vi "Time Countdown BAP4B.vi"(0 "Before Loop":i64, 1 "system state in":T1={"last light state"=enum."init", "light state"=enum."init", "state time (ms)"=0, "current time (ms)"=0, "time remaining (ms)"=0, "change state"=TRUE}, 3 "After  Loop":i64) -> (6 "system state out":T1={"last light state"=enum."init", "light state"=enum."init", "state time (ms)"=0, "current time (ms)"=0, "time remaining (ms)"=10000, "change state"=FALSE}, 9 "Timeout":bool)   [LabVIEW 2014]
doc: "Time Countdown BAP4B\n\nCounts down the current, remaining, and state time. If state time equals negative one, then there is unlimted remaining time, otherwise remaining time is less than state time, but greater than zero. Once reaching zero, it indicates to change state.\n\nBeverly Abadines\nPHY 350\nP4"
uses:
  typedefs/system state cluster.ctl
  typedefs/state enum.ctl
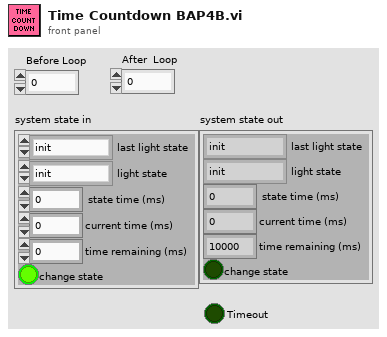
[diagram p1: front panel]
types:
  T1 = typedef "system state cluster.ctl" = cluster{"last light state":T2, "light state":T2, "state time (ms)":i32, "current time (ms)":i32, "time remaining (ms)":i32, "change state":bool}
  T2 = typedef "state enum.ctl" = enum16{"init", "idle", "left turn E", "go EW", "caution EW", "left turn W", "left turn N", "go NS", "caution NS", "left turn S", "blink on", "blink off", "all on test", "exit"}
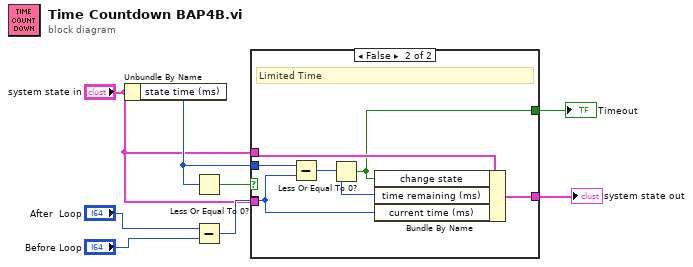
[diagram p0: block diagram]
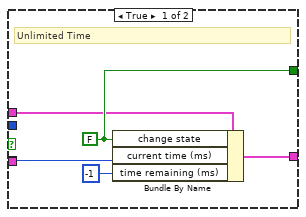
[diagram p2: hidden frame]
diagram:
  n1 = Unbundle By Name("system state in") -> ("state time (ms)"=w4:i32)
  n2 = Less Or Equal To 0?(x=w4) -> (x <= 0?=w5:bool)
  n3 = Subtract(x="After  Loop", y="Before Loop") -> (x-y=w6:i64)
  n4 = case shown="False" w5 {
    tunnel: w6 -> [w12 w16]
    tunnel: w4 -> [_ w18]
    tunnel: [w10 w14] -> w3
    tunnel: [w11 w17] -> w2
    tunnel: "system state in" -> [_ _]
    tunnel: "system state in" -> [w9 w15]
    frame True {
      w10 = FALSE
      # "Unlimited Time"
      n5 = Bundle By Name(cluster=w9, "change state"=w10, "current time (ms)"=w12, "time remaining (ms)"=-1) -> (w11:T1)
    }
    frame False {
      # "Limited Time"
      n6 = Subtract(x=w18, y=w16) -> (x-y=w19:i64)
      n7 = Less Or Equal To 0?(x=w19) -> (x <= 0?=w14:bool)
      n8 = Bundle By Name(cluster=w15, "change state"=w14, "time remaining (ms)"=w19, "current time (ms)"=w16) -> (w17:T1)
    }
  }
  "system state out" <- w2
  "Timeout" <- w3
